vi "NAND logic gates.vi"() -> ()   [LabVIEW 2010]
panel:
  out "NAND":bool
  in  "?":bool
  in  "?":bool
  out "NOR":bool
  in  "?":bool
  in  "?":bool
  in  "?":bool
  in  "?":bool
  out "XOR":bool
  in  "?":bool
  in  "?":bool
  out "NXOR":bool
  out "OR":bool
  in  "?":bool
  in  "?":bool
  in  "?":bool
  in  "?":bool
  out "AND":bool
  out "NOT":bool
  in  "?":bool
  # "Demonstration of Logic Gates composed of NAND gates."
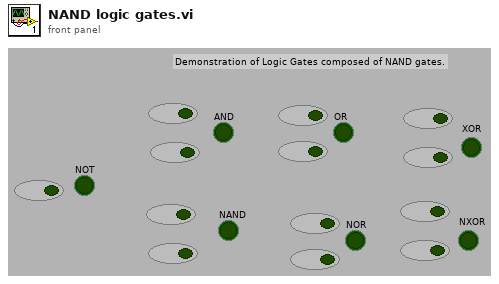
[diagram p1: front panel]
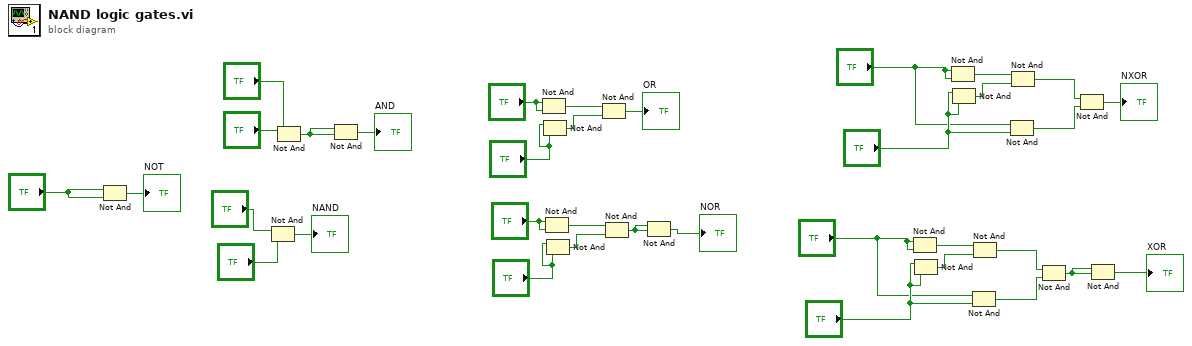
[diagram p0: block diagram]
diagram:
  n1 = Not And(1:"?", 2:"?") -> (0:→"NOT":bool)
  n2 = Not And(1:"?", 2:"?") -> (0:→"NAND":bool)
  n3 = Not And(1:"?", 2:"?") -> (0:w32:bool)
  n4 = Not And(1:w32, 2:w32) -> (0:→"AND":bool)
  n5 = Not And(1:"?", 2:"?") -> (0:w29:bool)
  n6 = Not And(1:"?", 2:"?") -> (0:w28:bool)
  n7 = Not And(1:"?", 2:"?") -> (0:w9:bool)
  n8 = Not And(1:"?", 2:"?") -> (0:w8:bool)
  n9 = Not And(1:w28, 2:w29) -> (0:→"OR":bool)
  n10 = Not And(1:w8, 2:w9) -> (0:w5:bool)
  n11 = Not And(1:w5, 2:w5) -> (0:→"NOR":bool)
  n12 = Not And(1:"?", 2:"?") -> (0:w17:bool)
  n13 = Not And(1:"?", 2:"?") -> (0:w16:bool)
  n14 = Not And(1:"?", 2:"?") -> (0:w24:bool)
  n15 = Not And(1:"?", 2:"?") -> (0:w23:bool)
  n16 = Not And(1:"?", 2:"?") -> (0:w14:bool)
  n17 = Not And(1:w16, 2:w17) -> (0:w15:bool)
  n18 = Not And(1:"?", 2:"?") -> (0:w21:bool)
  n19 = Not And(1:w23, 2:w24) -> (0:w22:bool)
  n20 = Not And(1:w14, 2:w15) -> (0:w11:bool)
  n21 = Not And(1:w21, 2:w22) -> (0:→"NXOR":bool)
  n22 = Not And(1:w11, 2:w11) -> (0:→"XOR":bool)
